vi "set control position Y.vi"(8 "error in (no error)":errorcluster, 10 "Top":i32, 11 "Control in":refnum<class "Control.lvclass">) -> (0 "error out":errorcluster, 3 "Control out":refnum<class "Control.lvclass">)   [LabVIEW 2010, in "Control.lvclass"]
uses:
  Control.lvclass
  Control.lvclass/Control.ctl
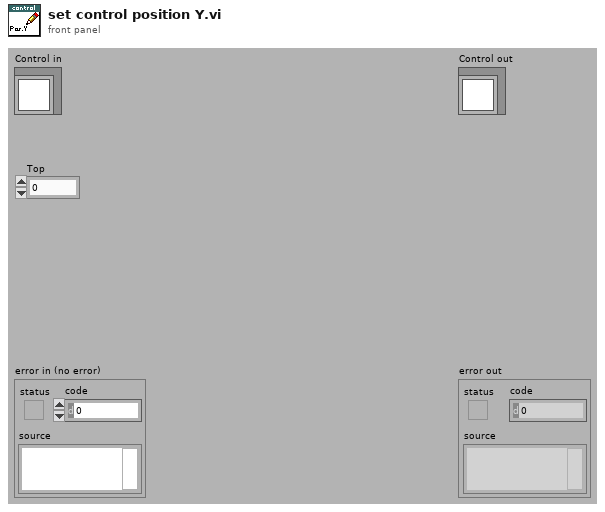
[diagram p1: front panel]
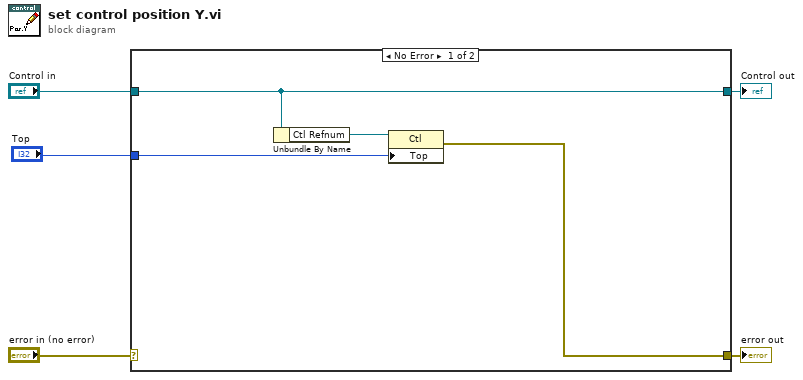
[diagram p0: block diagram]
diagram:
  n1 = case shown="No Error" "error in (no error)" {
    selector: "error in (no error)" -> [_ w11]
    tunnel: [w7 w11] -> w4
    tunnel: [w9 w10] -> w2
    tunnel: "Control in" -> [w9 w10]
    tunnel: "Top" -> [w6 _]
    frame No Error {
      n2 = Unbundle By Name(w9) -> ("Ctl Refnum"=w8:refnum<vi>)
      n3 = property class="Ctl"(reference=w8, "Top"=w6) -> (error out=w7:errorcluster)  [unwired: 1 in, 1 out]
    }
    frame Error {
    }
  }
  "error out" <- w4
  "Control out" <- w2
